vi "Build Messgenger.vi"(4 "Paras In 2":variant, 6 "Paras In":variant, 7 "Messenger Factory in":refnum<class "Messenger Factory.lvclass">, 8 "error in (no error)":errorcluster, 10 "Root Actor In":refnum<class "Root Actor.lvclass">, 11 "System Modules Factory In":refnum<class "System Modules Factory.lvclass">) -> (0 "error out":errorcluster, 2 "Root Actor Out":refnum<class "Root Actor.lvclass">, 3 "System Modules Factory Out":refnum<class "System Modules Factory.lvclass">, 5 "Messenger Factory out":refnum<class "Messenger Factory.lvclass">)   [LabVIEW 2024, in "Messenger Factory.lvclass"]
uses:
  Messenger Factory.lvclass
  Actor/Root Actor/Root Actor.lvclass
  System Modules Factory/System Modules Factory.lvclass
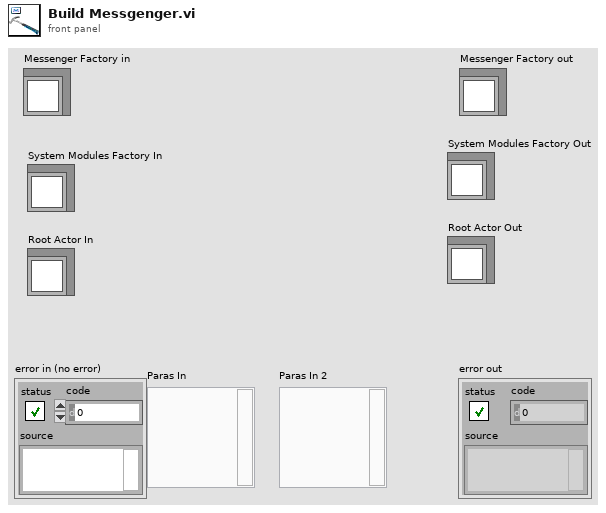
[diagram p1: front panel]
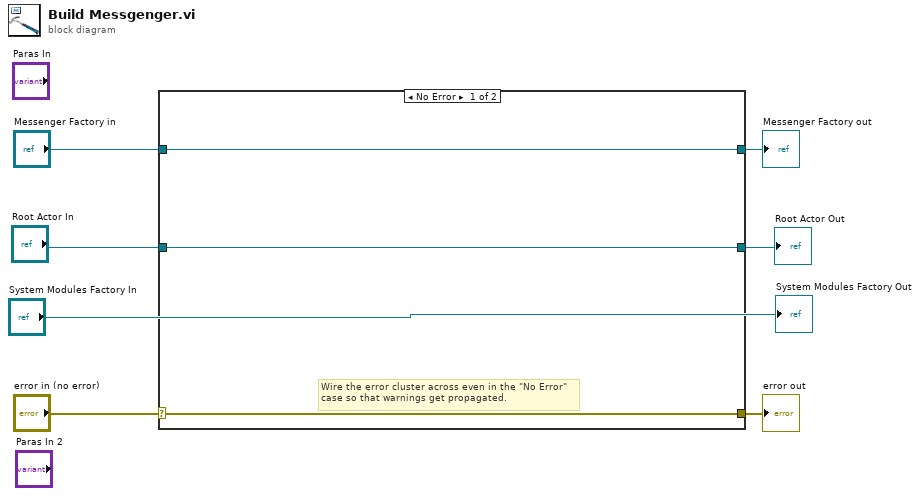
[diagram p0: block diagram]
diagram:
  n1 = case shown="No Error" "error in (no error)" {
    selector: "error in (no error)" -> [w9 w13]
    tunnel: [w9 w13] -> w6
    tunnel: [w10 w12] -> w4
    tunnel: "Messenger Factory in" -> [w10 w12]
    tunnel: [w8 w11] -> w2
    tunnel: "Root Actor In" -> [w8 w11]
    frame No Error {
      # "Wire the error cluster across even in the \"No Error\"\ncase so that warnings get propagated."
    }
    frame Error {
    }
  }
  "error out" <- w6
  "Messenger Factory out" <- w4
  "Root Actor Out" <- w2
  "System Modules Factory Out" <- "System Modules Factory In"
